vi "draw crosshairs.vi"(4 "color(black)":u32(colorbox), 6 "pen":T1={"Width"=1, "Style"=enum."Solid"}, 8 "Y":dbl, 9 "X":dbl, 10 "Rectangle":T2, 11 "picture":picture) -> (3 "new picture":picture)   [LabVIEW 2011]
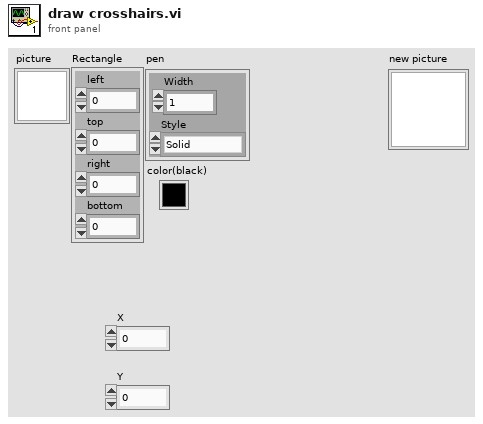
[diagram p1: front panel]
types:
  T1 = cluster{"Width":u16, "Style":enum32{"Solid", "Dash", "Dot", "DashDot", "DashDotDot"}}
  T2 = cluster{"left":i16, "top":i16, "right":i16, "bottom":i16}
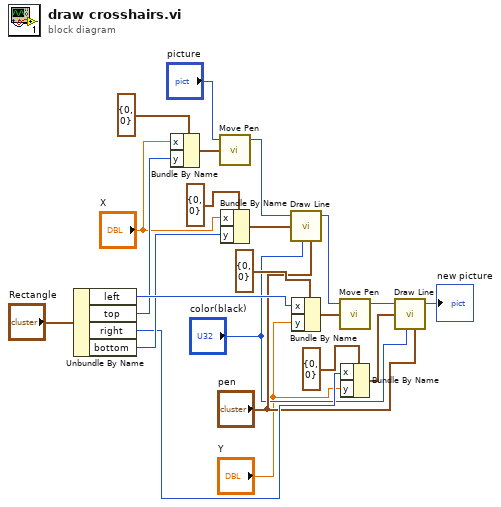
[diagram p0: block diagram]
diagram:
  n1 = Unbundle By Name("Rectangle") -> ("left"=w10:i16, "top"=w8:i16, "right"=w5:i16, "bottom"=w9:i16)
  n2 = Bundle By Name(cluster=cluster{"x":i16, "y":i16} {"x"=0, "y"=0} ("new position"), "x"="X", "y"=w8) -> (w15:cluster{"x":i16, "y":i16})
  n3 = call <vilib>:"Move Pen.vi"("new position"=w15, "picture"="picture") -> ("new picture"=w21:picture)  [unwired: 3 in]
  n4 = Bundle By Name(cluster=cluster{"x":i16, "y":i16} {"x"=0, "y"=0} ("new position"), "x"="X", "y"=w9) -> (w14:cluster{"x":i16, "y":i16})
  n5 = call <vilib>:"Draw Line.vi"("picture"=w21, "end point"=w14, "color(black)"="color(black)", "pen"="pen") -> ("new picture"=w18:picture)  [unwired: 5 in]
  n6 = Bundle By Name(cluster=cluster{"x":i16, "y":i16} {"x"=0, "y"=0} ("new position"), "x"=w10, "y"="Y") -> (w12:cluster{"x":i16, "y":i16})
  n7 = call <vilib>:"Move Pen.vi"("new position"=w12, "picture"=w18) -> ("new picture"=w20:picture)  [unwired: 3 in]
  n8 = Bundle By Name(cluster=cluster{"x":i16, "y":i16} {"x"=0, "y"=0} ("new position"), "x"=w5, "y"="Y") -> (w6:cluster{"x":i16, "y":i16})
  n9 = call <vilib>:"Draw Line.vi"("picture"=w20, "end point"=w6, "color(black)"="color(black)", "pen"="pen") -> ("new picture"=→"new picture":picture)  [unwired: 5 in]
